vi "Get Target IP Address2.vi"(8 "error in (no error)":errorcluster, 11 "SDF path":path) -> (0 "error out":errorcluster, 2 "target ip address":string)   [LabVIEW 2019, in "TimingDRV System Explorer.lvlib"]
uses:
  TimingDRV System Explorer.lvlib
  NationalInstruments.VeriStand.SystemDefinitionAPI
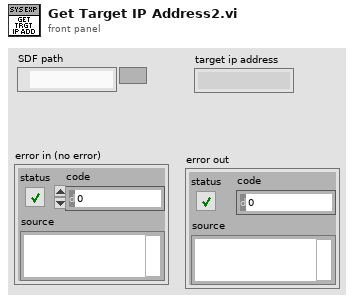
[diagram p1: front panel]
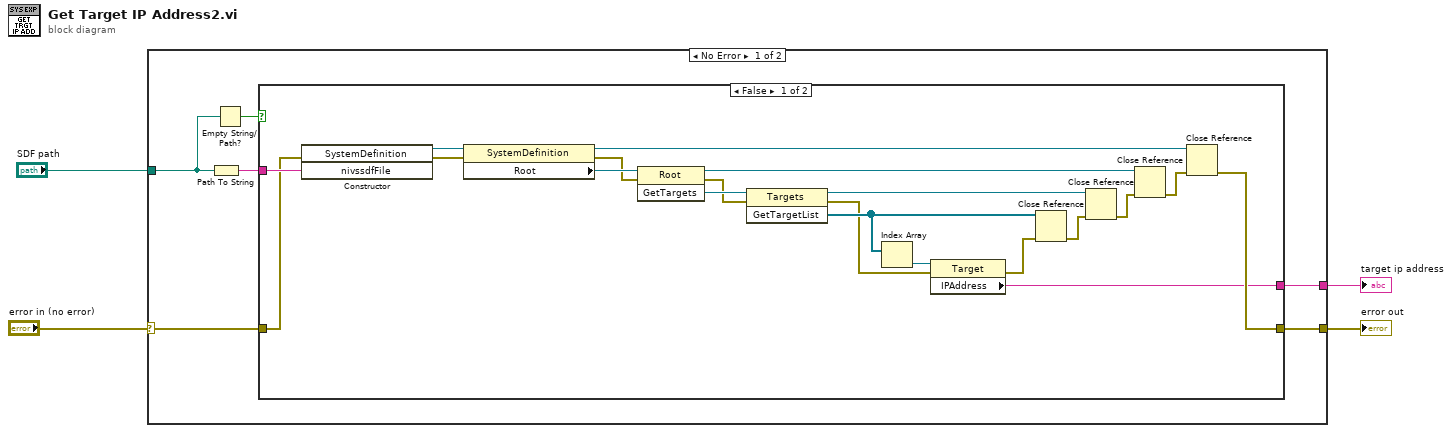
[diagram p0: block diagram]
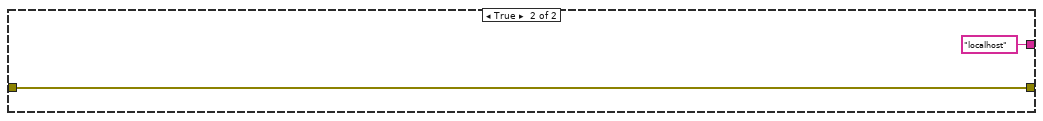
[diagram p2: hidden frame]
diagram:
  n1 = case shown="No Error" "error in (no error)" {
    selector: "error in (no error)" -> [w9 w33]
    tunnel: "SDF path" -> [w6 _]
    tunnel: [w8 w33] -> w1
    tunnel: [w7 _] -> w2
    frame No Error {
      n2 = Path To String(path=w6) -> (string=w10:string)
      n3 = Empty String/Path?(string/path=w6) -> (empty?=w5:bool)
      n4 = case shown="False" w5 {
        tunnel: w10 -> [w26 _]
        tunnel: w9 -> [w21 w31]
        tunnel: [w12 w31] -> w8
        tunnel: [w11 "localhost" ("IPAddress")] -> w7
        frame False {
          n5 = constructor class="SystemDefinition"(error in=w21, "nivssdfFile"=w26) -> (reference out=w27:refnum<k24>, error out=w20:errorcluster)  [unwired: 2 in, 2 out]
          n6 = property class="SystemDefinition"(reference=w27, error in=w20) -> (reference out=w25:refnum<k24>, error out=w19:errorcluster, "Root"=w28:refnum<k24>)
          n7 = invoke class="Root" method="GetTargets"(reference=w28, error in=w19) -> (reference out=w24:refnum<k24>, error out=w18:errorcluster, "GetTargets"=w29:refnum<k24>)  [unwired: 1 in]
          n8 = invoke class="Targets" method="GetTargetList"(reference=w29, error in=w18) -> (reference out=w23:refnum<k24>, error out=w17:errorcluster, "GetTargetList"=w22:refnum<k24>[])  [unwired: 1 in]
          n9 = Index Array(array=w22) -> (element=w30:refnum<k24>)  [unwired: 1 in]
          n10 = property class="Target"(reference=w30, error in=w17) -> (error out=w16:errorcluster, "IPAddress"=w11:string)  [unwired: 1 out]
          n11 = Close Reference(reference=w22, error in (no error)=w16) -> (error out=w15:errorcluster)
          n12 = Close Reference(reference=w23, error in (no error)=w15) -> (error out=w14:errorcluster)
          n13 = Close Reference(reference=w24, error in (no error)=w14) -> (error out=w13:errorcluster)
          n14 = Close Reference(reference=w25, error in (no error)=w13) -> (error out=w12:errorcluster)
        }
        frame True {
        }
      }
    }
    frame Error {
    }
  }
  "target ip address" <- w2
  "error out" <- w1
